vi "Expired.vi"(7 "Buffer (10 S)":dbl=10.0, 11 "Authorization in":refnum<class "Authorization.lvclass">) -> (2 "Expiry":T1)   [LabVIEW 2020, in "OAuth2.lvlib" / "Authorization.lvclass"]
uses:
  Authorization.lvclass
  Expiry.ctl
  Authorization.lvclass/Authorization.ctl
  OAuth2.lvlib
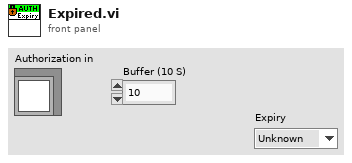
[diagram p1: front panel]
types:
  T1 = typedef "OAuth2.lvlib/Expiry.ctl" = enum16{"Unknown", "Expired", "Good"}
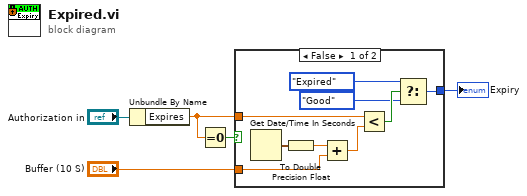
[diagram p0: block diagram]
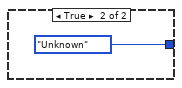
[diagram p2: hidden frame]
diagram:
  n1 = Unbundle By Name("Authorization in") -> ("Expires"=w2:dbl)
  n2 = Equal To 0?(x=w2) -> (x = 0?=w4:bool)
  n3 = case shown="False" w4 {
    tunnel: [w6 Expiry."Unknown" ("Expiry")] -> w3
    tunnel: w2 -> [w11 _]
    tunnel: "Buffer (10 S)" -> [w13 _]
    frame False {
      n4 = Get Date/Time In Seconds() -> (seconds since 1Jan1904=w14:timestamp)
      n5 = To Double Precision Float(number=w14) -> (double precision float=w12:dbl)
      n6 = Add(x=w12, y=w13) -> (x+y=w10:dbl)
      n7 = Less?(x=w11, y=w10) -> (x < y?=w9:bool)
      n8 = Select(t=Expiry."Expired" ("Expiry"), s=w9, f=Expiry."Good" ("Expiry")) -> (s? t:f=w6:T1)
    }
    frame True {
    }
  }
  "Expiry" <- w3
